vi "TX_Couping(DEBUG).vi"() -> ()   [LabVIEW 2015]
uses:
  <instrlib>/Rohde&Schwarz Spectrum Analyzer/Rohde&Schwarz Spectrum Analyzer.lvlib
panel:
  in  "A-B/B-A":enum16{"B2A", "A2B"}(ring)
  in  "O_R&S Spec1 2":refnum<visa-resource-name>
  in  "O_R&S Spec1":refnum<visa-resource-name>="GPIB0::22::INSTR"
  out "B通道发射带":cluster{"X":dbl[], "Amplitude":dbl[]}(graph)
  out "A通道发射带":cluster{"X":dbl[], "Amplitude":dbl[]}(graph)
  in  "发射带末频率(Mhz)":u32=2130 caption="Start Frequency (0.0)"
  in  "发射带始频率(Mhz)":u32=2018 caption="Stop Frequency (0.0)"
  out "B_peak":dbl[](array[numeric])
  out "B_pos":dbl[](array[numeric])
  out "Array 6":cluster{"X":dbl[], "Amplitude":dbl[]}[](array[cluster])
  out "A_peak":dbl[](array[numeric])
  out "A_pos":dbl[](array[numeric])
  out "Array":cluster{"X":dbl[], "Amplitude":dbl[]}[](array[cluster])
  in  "OK":bool
  in  "stop":bool
  out "Bx":dbl[](array[numeric]) caption="X" format="%^.3e"
  out "By":dbl[](array[numeric]) caption="Amplitude" format="%^.3e"
  out "B_pos":dbl caption="Marker Position" format="%^.3e"
  out "B_peak":dbl caption="Marker Amplitude" format="%^.3e"
  out "A_peak":dbl caption="Marker Amplitude" format="%^.3e"
  out "A_pos":dbl caption="Marker Position" format="%^.3e"
  out "Ay":dbl[](array[numeric]) caption="Amplitude" format="%^.3e"
  out "Ax":dbl[](array[numeric]) caption="X" format="%^.3e"
  in  "VISA resource name 2":refnum<visa-resource-name>="COM3"
  out "Freq_Tab":u32[](array[numeric])
  in  "Insert Point":u32
  in  "EABLE Insert":bool
  in  "Value":u32=10 caption="Point Num"
  in  "cnt/setp":enum16{"SETP", "COUNT"}(ring)=enum."COUNT"
  in  "freq_max(Mhz)":u32=2123
  in  "freq_min(Mhz)":u32=2018
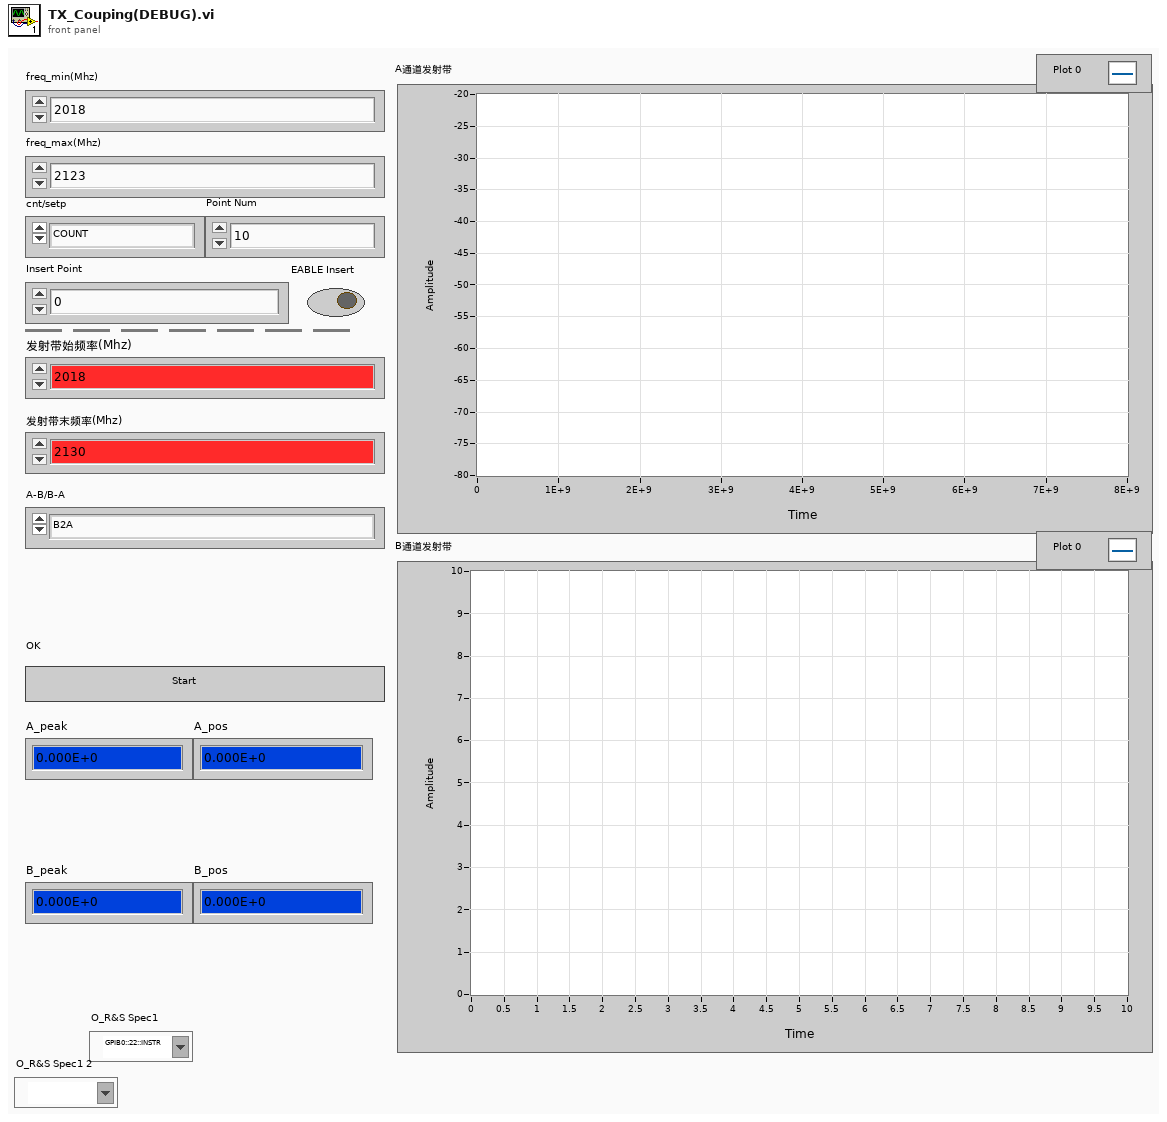
[diagram p1: front panel]
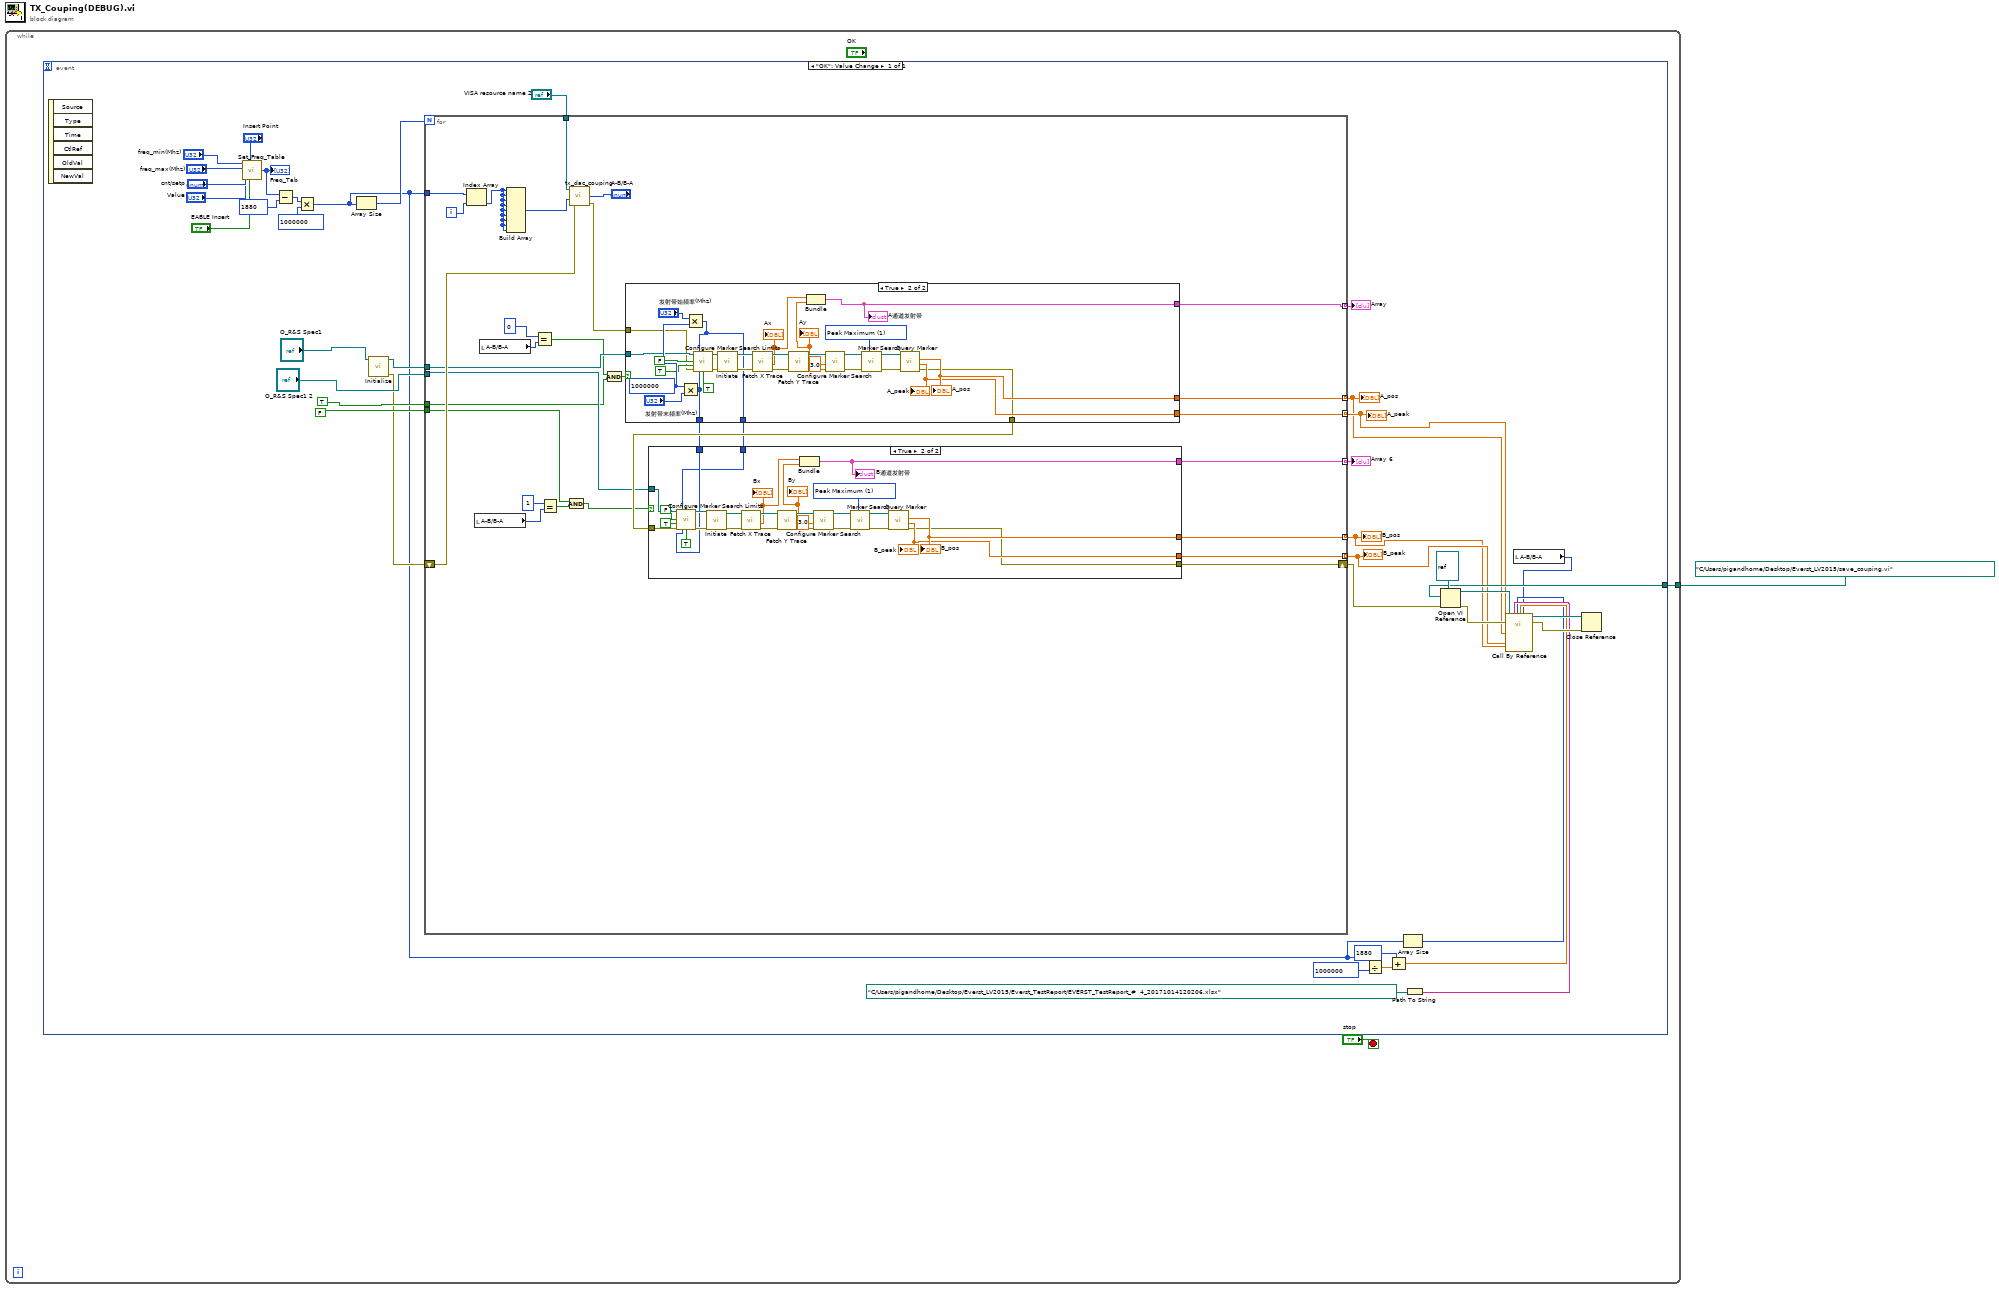
[diagram p0: block diagram]
diagram:
  n1 = while {
    tunnel: path "C:/Users/pigandhome/Desktop/Everst_LV2015/save_couping.vi" ("vi path") -> [w2]
    stop <- "stop" stop-if-true
    n2 = event shown="[0] \"OK\": Value Change" {
      selector: _ -> [_]
      dyn-events: _ -> [_]
      timeout: _ -> [_]
      tunnel: w2 -> [w23]
      event "OK": Value Change {
        n3 = event-data() -> ()  [unwired: 1 in, 6 out]
        n4 = call "Set_Freq_Table.vi"("EABLE Insert"="EABLE Insert", "Insert Point"="Insert Point", "Value"="Value", "cnt/setp"="cnt/setp", "freq_max(Mhz)"="freq_max(Mhz)", "freq_min(Mhz)"="freq_min(Mhz)") -> ("Freq_Tab"=w37:u32[])
        "Freq_Tab" <- w37
        n5 = Subtract(x=w37, y=1880) -> (x-y=w35:u32[])
        n6 = Multiply(x=w35, y=1000000) -> (x*y=w6:u32[])
        n7 = Array Size(array=w6) -> (size(s)=w33:i32)
        n8 = call <instrlib>:"Initialize.vi"("VISA resource name"="O_R&S Spec1") -> ("VISA resource name out"=w17:refnum<visa-resource-name>, "error out"=w15:errorcluster)  [unwired: 13 in]
        n9 = for {
          N: w33 -> [_]
          tunnel: w6 -> [w72]
          tunnel: "VISA resource name 2" -> [w71]
          tunnel: w17 -> [w59]
          tunnel: "O_R&S Spec1 2" -> [w58]
          tunnel: TRUE ("spec1_state") -> [w45]
          tunnel: FALSE ("spec1_state") -> [w47]
          shift-right: [w57] -> w24
          shift-left: w15 -> [w67]
          tunnel: [w65] -> w9 mode=indexing
          tunnel: [w64] -> w10 mode=indexing
          tunnel: [w63] -> w7 mode=indexing
          tunnel: [w62] -> w8 mode=indexing
          tunnel: [w61] -> w31 mode=indexing
          tunnel: [w60] -> w30 mode=indexing
          i -> [w73]
          n10 = Index Array(array=w72, index=w73) -> (element=w66:u32)
          n11 = local read "A-B/B-A"() -> (w49:enum16{"B2A", "A2B"})
          n12 = local read "A-B/B-A"() -> (w52:enum16{"B2A", "A2B"})
          n13 = Build Array(w66, w66, w66, w66, w66, w66, w66, w66, w66) -> (w70:u32[])
          n14 = Equal?(x=0, y=w52) -> (x = y?=w46:bool)
          n15 = Equal?(x=u32 1, y=w49) -> (x = y?=w48:bool)
          n16 = And(x=w47, y=w48) -> (x .and. y?=w44:bool)
          n17 = call "tx_dac_couping.vi"("Enum"="A-B/B-A", "error in (no error)"=w67, "fin"=w70, "VISA resource name 2"=w71) -> ("error out"=w69:errorcluster)  [unwired: 2 in]
          n18 = And(x=w46, y=w45) -> (x .and. y?=w53:bool)
          n19 = case shown="True" w53 {
            tunnel: w59 -> [_ w106]
            tunnel: w69 -> [w101 w105]
            tunnel: [w101 w104] -> w68
            tunnel: [_ w119] -> w65
            tunnel: [_ w118] -> w64
            tunnel: [_ w112] -> w61
            tunnel: [_ w103] -> w56
            tunnel: [_ w102] -> w55
            frame False {
            }
            frame True {
              w113 = u32 1000000 ("x")
              w120 = 1 items=["Peak Maximum"=1, "Peak Minimum"=2, "Next Maximum"=3, "Left Maximum"=4, "Right Maximum"=5, "Next Minimum"=6, "Left Minimum"=7, "Right Minimum"=8] ("Marker Search (Peak Maximum)")
              n20 = Multiply(x=w113, y="发射带末频率(Mhz)") -> (x*y=w103:u32)
              n21 = Multiply(x="发射带始频率(Mhz)", y=w113) -> (x*y=w102:u32)
              n22 = call <instrlib>:"Configure Marker Search Limits.vi"("VISA resource name"=w106, "Search Limit Left (0.0)"=w102, "Threshold State (T: On)"=FALSE, "Search Limits (F: Off)"=TRUE, "error in (no error)"=w105, "Search Limit Right (0.0)"=w103, "Search Limits Zoom (F: Off)"=TRUE) -> ("VISA resource name out"=w110:refnum<visa-resource-name>, "error out"=w111:errorcluster)  [unwired: 7 in]
              n23 = call <instrlib>:"Initiate.vi"("error in (no error)"=w111, "VISA resource name"=w110) -> ("error out"=w131:errorcluster, "VISA resource name out"=w130:refnum<visa-resource-name>)  [unwired: 8 in]
              n24 = call <instrlib>:"Fetch X Trace.vi"("error in (no error)"=w131, "VISA resource name"=w130) -> ("error out"=w129:errorcluster, "X"=w117:dbl[], "VISA resource name out"=w128:refnum<visa-resource-name>)  [unwired: 7 in]
              "Ax" <- w117
              n25 = call <instrlib>:"Fetch Y Trace.vi"("error in (no error)"=w129, "VISA resource name"=w128) -> ("error out"=w127:errorcluster, "Amplitude"=w116:dbl[], "VISA resource name out"=w126:refnum<visa-resource-name>)  [unwired: 7 in]
              "Ay" <- w116
              n26 = Bundle("X"=w117, "Amplitude"=w116) -> (w112:cluster{"X":dbl[], "Amplitude":dbl[]})  [unwired: 1 in]
              "A通道发射带" <- w112
              n27 = call <instrlib>:"Configure Marker Search.vi"("error in (no error)"=w127, "Peak Excursion (6.0)"=3.0, "VISA resource name"=w126) -> ("error out"=w125:errorcluster, "VISA resource name out"=w124:refnum<visa-resource-name>)  [unwired: 7 in]
              n28 = call <instrlib>:"Marker Search.vi"("Marker Search (Peak Maximum)"=w120, "error in (no error)"=w125, "VISA resource name"=w124) -> ("error out"=w123:errorcluster, "VISA resource name out"=w122:refnum<visa-resource-name>)  [unwired: 7 in]
              n29 = call <instrlib>:"Query Marker.vi"("error in (no error)"=w123, "VISA resource name"=w122) -> ("error out"=w104:errorcluster, "Marker Amplitude"=w118:dbl, "Marker Position"=w119:dbl)  [unwired: 6 in, 1 out]
              "A_pos" <- w119
              "A_peak" <- w118
            }
          }
          n30 = case shown="True" w44 {
            tunnel: w58 -> [_ w81]
            tunnel: w68 -> [w74 w88]
            tunnel: [w74 w82] -> w57
            tunnel: [_ w87] -> w63
            tunnel: [_ w86] -> w62
            tunnel: [_ w83] -> w60
            tunnel: w56 -> [_ w76]
            tunnel: w55 -> [_ w75]
            frame False {
            }
            frame True {
              w100 = 1 items=["Peak Maximum"=1, "Peak Minimum"=2, "Next Maximum"=3, "Left Maximum"=4, "Right Maximum"=5, "Next Minimum"=6, "Left Minimum"=7, "Right Minimum"=8] ("Marker Search (Peak Maximum)")
              n31 = call <instrlib>:"Configure Marker Search Limits.vi"("VISA resource name"=w81, "Search Limit Left (0.0)"=w75, "Threshold State (T: On)"=FALSE, "Search Limits (F: Off)"=TRUE, "Search Limit Right (0.0)"=w76, "Search Limits Zoom (F: Off)"=TRUE) -> ("VISA resource name out"=w80:refnum<visa-resource-name>)  [unwired: 8 in, 1 out]
              n32 = call <instrlib>:"Initiate.vi"("error in (no error)"=w88, "VISA resource name"=w80) -> ("error out"=w89:errorcluster, "VISA resource name out"=w90:refnum<visa-resource-name>)  [unwired: 8 in]
              n33 = call <instrlib>:"Fetch X Trace.vi"("error in (no error)"=w89, "VISA resource name"=w90) -> ("error out"=w91:errorcluster, "X"=w85:dbl[], "VISA resource name out"=w92:refnum<visa-resource-name>)  [unwired: 7 in]
              "Bx" <- w85
              n34 = call <instrlib>:"Fetch Y Trace.vi"("error in (no error)"=w91, "VISA resource name"=w92) -> ("error out"=w93:errorcluster, "Amplitude"=w84:dbl[], "VISA resource name out"=w94:refnum<visa-resource-name>)  [unwired: 7 in]
              "By" <- w84
              n35 = Bundle("X"=w85, "Amplitude"=w84) -> (w83:cluster{"X":dbl[], "Amplitude":dbl[]})  [unwired: 1 in]
              "B通道发射带" <- w83
              n36 = call <instrlib>:"Configure Marker Search.vi"("error in (no error)"=w93, "Peak Excursion (6.0)"=3.0, "VISA resource name"=w94) -> ("error out"=w95:errorcluster, "VISA resource name out"=w96:refnum<visa-resource-name>)  [unwired: 7 in]
              n37 = call <instrlib>:"Marker Search.vi"("Marker Search (Peak Maximum)"=w100, "error in (no error)"=w95, "VISA resource name"=w96) -> ("error out"=w97:errorcluster, "VISA resource name out"=w98:refnum<visa-resource-name>)  [unwired: 7 in]
              n38 = call <instrlib>:"Query Marker.vi"("error in (no error)"=w97, "VISA resource name"=w98) -> ("error out"=w82:errorcluster, "Marker Amplitude"=w86:dbl, "Marker Position"=w87:dbl)  [unwired: 6 in, 1 out]
              "B_pos" <- w87
              "B_peak" <- w86
            }
          }
        }
        "Array" <- w31
        "A_pos" <- w9
        "A_peak" <- w10
        "Array 6" <- w30
        "B_pos" <- w7
        "B_peak" <- w8
        n39 = Divide(x=w6, y=u32 1000000) -> (x/y=w13:dbl[])
        n40 = Add(x=u32 1880, y=w13) -> (x+y=w11:dbl[])
        n41 = Array Size(array=w6) -> (size(s)=w5:i32)
        n42 = Path To String(path=path "C:/Users/pigandhome/Desktop/Everst_LV2015/Everst_TestReport/EVERST_TestReport_#  4_20171014120206.xlsx") -> (string=w22:string)
        n43 = Open VI Reference(type specifier VI Refnum (for type only)=refnum<vi> refnum, vi path=w23, error in (no error)=w24) -> (vi reference=w29:refnum<vi>, error out=w28:errorcluster)  [unwired: 3 in]
        n44 = local read "A-B/B-A"() -> (w4:enum16{"B2A", "A2B"})
        n45 = call-by-ref "?"(reference=w29, error in=w28, "Apeak"=w10, "Apeakpos"=w9, "Bpeak"=w8, "Bpeakpos"=w7, "PATH"=w22, "Tabsize"=w5, "FreqTab"=w11, "MODE"=w4) -> (reference out=w25:refnum<vi>, error out=w26:errorcluster)  [unwired: 12 in]
        n46 = Close Reference(reference=w25, error in (no error)=w26) -> ()  [unwired: 1 out]
      }
    }
  }
